vi "CreateCaptureFileName.vi"(10 "OOB to Logic Data out":T1 {"ExportType" items=["PNG", "RAW"]}, 11 "image metadata":T3={"serial channel"=0.0, "frame number"=0, "data type"=enum."Frame Start", "width"=0, "height"=0, "image bytes"=0, "total bytes"=0, "little endian"=FALSE, "Status"="Ready for Acquisition"}) -> (3 "Path":path)   [LabVIEW 2025, in "Automotive Vision.lvclass"]
uses:
  <instrlib>/FlexRIO/CSI-2/v2/Common/Types/LLP Data Type.ctl
  Automotive-Vision OOB Data Transfer/Typdefs/OOB to Logic Data.ctl
  Automotive Vision.lvclass
  Automotive Vision.lvclass/Automotive Vision.ctl
  <instrlib>/FlexRIO/CSI-2/v2/Common/NI CSI-2 API Common v2.lvlib
  Automotive-Vision OOB Data Transfer/Automotive-Vision OOB Data Transfer.lvlib
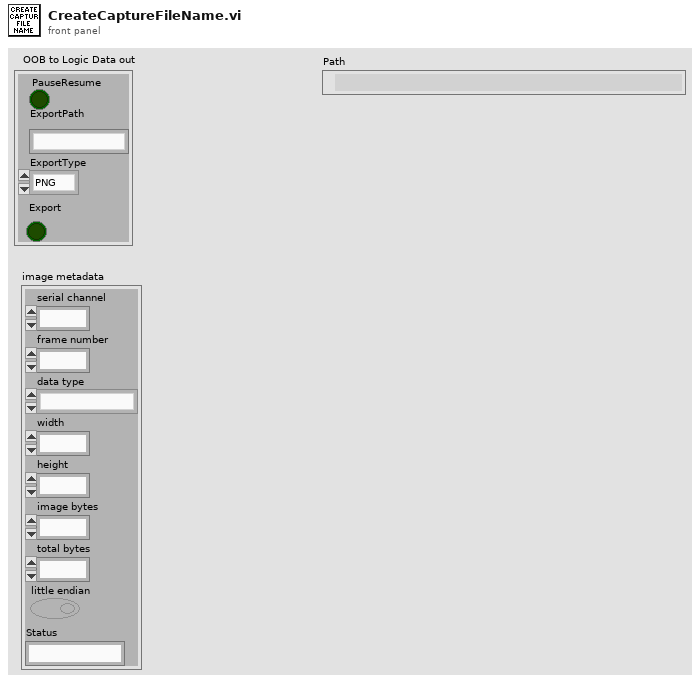
[diagram p1: front panel]
types:
  T1 = typedef "Automotive-Vision OOB Data Transfer.lvlib/OOB to Logic Data.ctl" = cluster{"PauseResume":bool, "ExportPath":string, "ExportType":u16, "Export":bool}
  T2 = typedef "NI CSI-2 API Common v2.lvlib/LLP Data Type.ctl" = enum8{"Frame Start", "Frame End", "Line Start", "Line End", "End of Transmission", "Reserved 0", "Reserved 1", "Reserved 2", "Generic Short Packet 1", "Generic Short Packet 2", "Generic Short Packet 3", "Generic Short Packet 4", "Generic Short Packet 5", "Generic Short Packet 6", "Generic Short Packet 7", "Generic Short Packet 8", "Null", "Blanking Data", "Embedded 8-bit non Image Data", "Generic Long Packet 1", "Generic Long Packet 2", "Generic Long Packet 3", "Generic Long Packet 4", "Reserved 3", "YUV420 8-bit", "YUV420 10-bit", "Legacy YUV420 8-bit", "Reserved 4", "YUV420 8-bit Chroma Shifted", "YUV420 10-bit Chroma Shifted", "YUV422 8-bit", "YUV422 10-bit", "RGB444", "RGB555", "RGB565", "RGB666", "RGB888", "Reserved 5", "Reserved 6", "RAW 24", "RAW 6", "RAW 7", "RAW 8", "RAW 10", "RAW 12", "RAW 14", "RAW 16", "RAW 20", "User Defined 8-bit Data 1", "User Defined 8-bit Data 2", "User Defined 8-bit Data 3", "User Defined 8-bit Data 4", "User Defined 8-bit Data 5", "User Defined 8-bit Data 6", "User Defined 8-bit Data 7", "User Defined 8-bit Data 8", "USL Command", "Reserved 7", "Reserved 8", "Reserved 9", "Reserved 10", "Reserved 11", "Reserved 12", "LRTE EPD Spacer"}
  T3 = cluster{"serial channel":fxp<+,3,3>, "frame number":u16, "data type":T2, "width":u16, "height":u16, "image bytes":u32, "total bytes":u32, "little endian":bool, "Status":string}
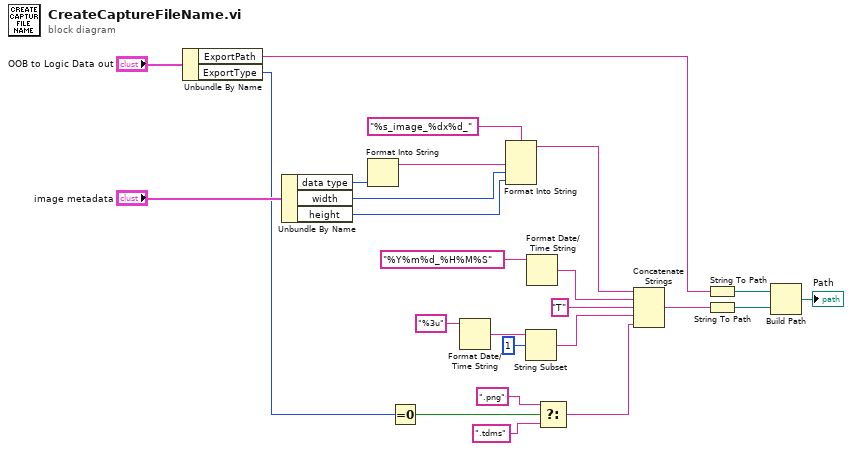
[diagram p0: block diagram]
diagram:
  n1 = Unbundle By Name("OOB to Logic Data out") -> ("ExportPath"=w6:string, "ExportType"=w3:u16)
  n2 = Unbundle By Name("image metadata") -> ("data type"=w17:T2, "width"=w14:u16, "height"=w13:u16)
  n3 = Format Into String(w17) -> (resulting string=w15:string)  [unwired: 3 in, 1 out]
  n4 = Equal To 0?(x=w3) -> (x = 0?=w2:bool)
  n5 = Format Date/Time String(time format string (%c)="%3u") -> (date/time string=w21:string)  [unwired: 2 in]
  n6 = Format Into String(format string="%s_image_%dx%d_" ("time format string (%c)"), w15, w14, w13) -> (resulting string=w12:string)  [unwired: 2 in, 1 out]
  n7 = String Subset(string=w21, offset (0)=1) -> (substring=w19:string)  [unwired: 1 in]
  n8 = Format Date/Time String(time format string (%c)="%Y%m%d_%H%M%S") -> (date/time string=w22:string)  [unwired: 2 in]
  n9 = Select(t=".png" ("string"), s=w2, f=".tdms" ("string")) -> (s? t:f=w1:string)
  n10 = Concatenate Strings(w12, w22, "T" ("string"), w19, w1) -> (w10:string)
  n11 = String To Path(string=w6) -> (path=w8:path)
  n12 = String To Path(string=w10) -> (path=w9:path)
  n13 = Build Path(base path=w8, name or relative path=w9) -> (appended path=→"Path":path)
